vi "InitDMA.vi"(8 "error in (no error)":errorcluster, 11 "FpgaRef5761 in":refnum<class "FpgaRef5761.lvclass">) -> (0 "error out":errorcluster, 3 "FpgaRef5761 out":refnum<class "FpgaRef5761.lvclass">)   [LabVIEW 2018, in "FpgaRef5761.lvclass"]
uses:
  FpgaRef5761.lvclass
  FpgaRef5761.lvclass/FpgaRef5761.ctl
  <vilib>/rvi/interface/common/niFpgaWaitOnOcc.vi
  <vilib>/Utility/error.llb/Error Cluster From Error Code.vi
  <vilib>/rvi/errors/niLvFpgaAdjustHostInterfaceError.vi
  <vilib>/rvi/interface/nirviMethod/nirviMethod.xnode
  5761 FPGA ref.ctl
  <vilib>/FPGAPlugInAG/Dynamic/niLvFpga_StartFifo_Dynamic.vi
  <vilib>/rvi/errors/niLvFpgaMergeErrorWithErrorCode.vi
  <vilib>/FPGAPlugInAG/Dynamic/niLvFpga_ConfigureFifo_Dynamic.vi
  <vilib>/FPGAPlugInAG/Dynamic/niLvFpga_ReadFifo_Dynamic.vi
panel:
  out "Actual Depth":u32
  out "Remaining":u32
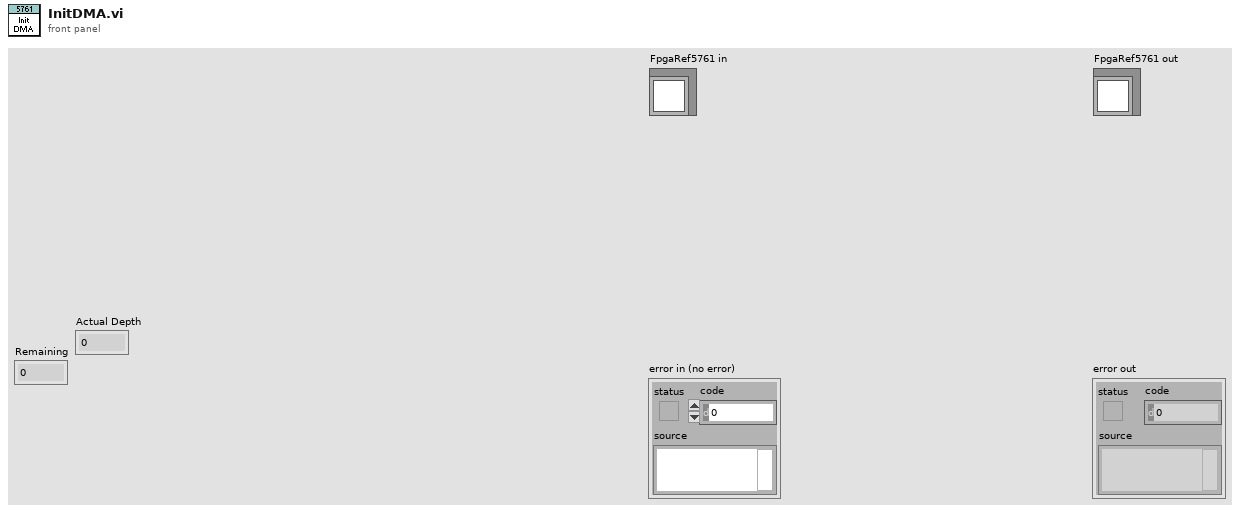
[diagram p1: front panel]
types:
  T1 = typedef "5761 FPGA ref.ctl" = refnum<k20>
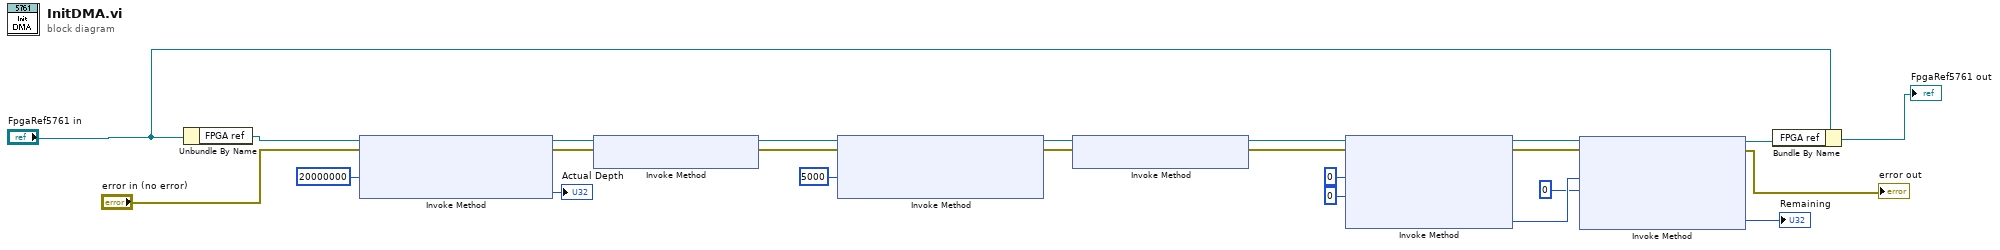
[diagram p0: block diagram]
diagram:
  n1 = Unbundle By Name("FpgaRef5761 in") -> ("FPGA ref"=w5:T1)
  n2 = xnode "Invoke Method"("FPGA VI Reference In"=w5, "error in"="error in (no error)", "Requested Depth"=u32 20000000 ("Depth")) -> ("FPGA VI Reference Out"=w22:T1, "error out"=w23:errorcluster, "Actual Depth"=→"Actual Depth":u32)
  n3 = xnode "Invoke Method"("FPGA VI Reference In"=w22, "error in"=w23) -> ("FPGA VI Reference Out"=w11:T1, "error out"=w10:errorcluster)
  n4 = xnode "Invoke Method"("FPGA VI Reference In"=w11, "error in"=w10, "Requested Depth"=u32 5000 ("Depth")) -> ("FPGA VI Reference Out"=w14:T1, "error out"=w13:errorcluster)  [unwired: 1 out]
  n5 = xnode "Invoke Method"("FPGA VI Reference In"=w14, "error in"=w13) -> ("FPGA VI Reference Out"=w8:T1, "error out"=w9:errorcluster)
  n6 = xnode "Invoke Method"("FPGA VI Reference In"=w8, "error in"=w9, "Number of Elements"=u32 0, "Timeout (ms)"=0) -> ("FPGA VI Reference Out"=w17:T1, "error out"=w16:errorcluster, "Elements Remaining"=w19:u32)  [unwired: 1 out]
  n7 = xnode "Invoke Method"("FPGA VI Reference In"=w17, "error in"=w16, "Number of Elements"=w19, "Timeout (ms)"=0) -> ("FPGA VI Reference Out"=w2:T1, "error out"=→"error out":errorcluster, "Elements Remaining"=→"Remaining":u32)  [unwired: 1 out]
  n8 = Bundle By Name(cluster="FpgaRef5761 in", "FPGA ref"=w2) -> (→"FpgaRef5761 out":refnum<class "FpgaRef5761.lvclass">)
